vi "Test MQTT-3.8.3-3.vi"(8 "error in (no error)":errorcluster) -> (0 "error out":errorcluster)   [LabVIEW 2013]
uses:
  source/Control Packets/SUBSCRIBE/Topic Subscription -- cluster.ctl
  source/Control Packets/ControlPacket/QualityOfService -- enum.ctl
  source/Control Packets/ControlPacket/ControlPacket.lvclass/ControlPacket.ctl
  source/Client/Client.lvclass
  <vilib>/addons/_JKI Toolkits/Caraya/classes/Test/Test.lvclass
  source/Control Packets/SUBSCRIBE/SUBSCRIBE.lvclass
  source/Control Packets/ControlPacket/ControlPacket.lvclass
  <vilib>/addons/_JKI Toolkits/Caraya/classes/Assert/Assert.lvclass
  source/MQTT_Base/MQTT_Base.lvclass
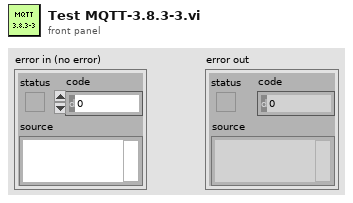
[diagram p1: front panel]
types:
  T1 = typedef "SUBSCRIBE.lvclass/Topic Subscription -- cluster.ctl" = cluster{"Topic Filter":string, "QoS":T2}
  T2 = typedef "ControlPacket.lvclass/QualityOfService -- enum.ctl" = enum16{"0 (At Most Once)", "1 (At Least Once)", "2 (Exactly Once)"}
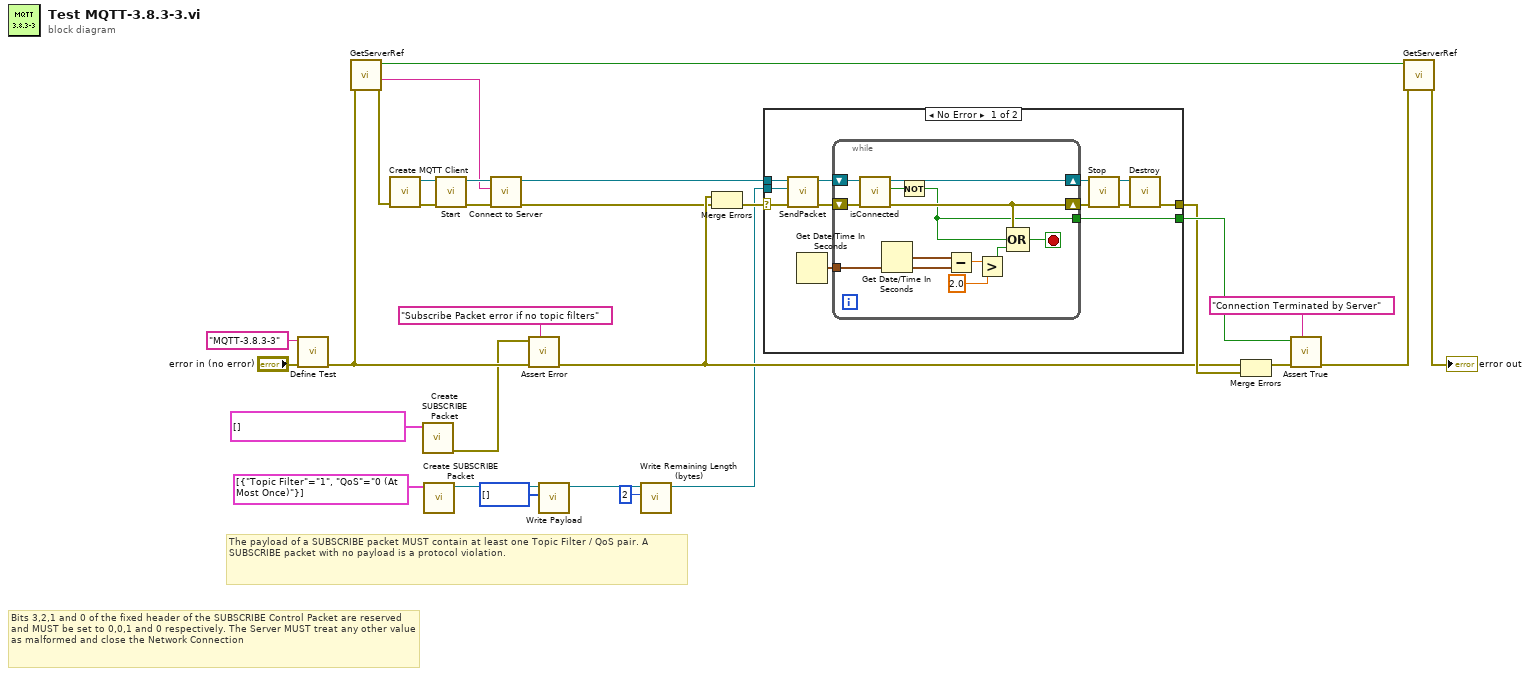
[diagram p0: block diagram]
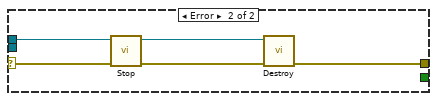
[diagram p2: hidden frame]
diagram:
  # "The payload of a SUBSCRIBE packet MUST contain at least one Topic Filter / QoS pair. A SUBSCRIBE packet with no payload is a protocol violation."
  # "Bits 3,2,1 and 0 of the fixed header of the SUBSCRIBE Control Packet are reserved and MUST be set to 0,0,1 and 0 respectively. The Server MUST treat any other value as malformed and close the Network Connection"
  n1 = call <vilib>:"Define Test.vi"("error in (no error)"="error in (no error)", "Label (VI Title)"="MQTT-3.8.3-3") -> ("error out"=w19:errorcluster)  [unwired: 9 in]
  n2 = call "GetServerRef.vi"("error in"=w19) -> ("error out"=w26:errorcluster, "Server address"=w1:string, "Created"=w27:bool)  [unwired: 7 in, 1 out]
  n3 = call "Create MQTT Client.vi"("error in (no error)"=w26) -> ("error out"=w10:errorcluster, "Client out"=w12:refnum<class "Client.lvclass">)  [unwired: 9 in]
  n4 = call "Create SUBSCRIBE Packet.vi"("Topic Subscriptions"=T1[] []) -> ("error out"=w8:errorcluster)  [unwired: 9 in, 1 out]
  n5 = call "Create SUBSCRIBE Packet.vi"("Topic Subscriptions"=T1[] [{"Topic Filter"="1", "QoS"=enum."0 (At Most Once)"}]) -> ("SUBSCRIBE out"=w6:refnum<class "SUBSCRIBE.lvclass">)  [unwired: 9 in, 1 out]
  n6 = call "Start.vi"("error in (no error)"=w10, "MQTT_Base in"=w12) -> ("error out"=w9:errorcluster, "MQTT_Base out"=w11:refnum<class "Client.lvclass">)  [unwired: 7 in, 1 out]
  n7 = call "Connect to Server.vi"("error in (no error)"=w9, "address (localhost)"=w1, "Client in"=w11) -> ("error out"=w14:errorcluster, "Client out"=w13:refnum<class "Client.lvclass">)  [unwired: 6 in, 1 out]
  n8 = call <vilib>:"Assert Error.vi"("Label"="Subscribe Packet error if no topic filters", "error in (no error)"=w19, "Error?"=w8) -> ("error out"=w16:errorcluster)  [unwired: 8 in]
  n9 = call "Write Payload.vi"("Payload"=u8[] [], "ControlPacket in"=w6) -> ("ControlPacket out"=w2:refnum<class "SUBSCRIBE.lvclass">)  [unwired: 9 in]
  n10 = call "Write Remaining Length (bytes).vi"("Remaining Length (bytes)"=u32 2, "ControlPacket in"=w2) -> ("ControlPacket out"=w4:refnum<class "SUBSCRIBE.lvclass">)  [unwired: 9 in]
  n11 = Merge Errors(w16, w14) -> (w15:errorcluster)
  n12 = case shown="No Error" w15 {
    selector: w15 -> [w39 w55]
    tunnel: w13 -> [w40 w57]
    tunnel: [w41 w58] -> w17
    tunnel: [w31 _] -> w22
    tunnel: w4 -> [w38 _]
    frame No Error {
      n13 = call "SendPacket.vi"("error in (no error)"=w39, "ControlPacket"=w38, "Client in"=w40) -> ("error out"=w34:errorcluster, "Client out"=w35:refnum<class "Client.lvclass">)  [unwired: 6 in, 1 out]
      n14 = Get Date/Time In Seconds() -> (seconds since 1Jan1904=w30:timestamp)
      n15 = while {
        shift-right: [w50] -> w33
        shift-left: w34 -> [w51]
        shift-right: [w52] -> w32
        shift-left: w35 -> [w53]
        tunnel: [w47] -> w31
        tunnel: w30 -> [w42]
        stop <- w49 stop-if-true
        n16 = call "isConnected.vi"("error in (no error)"=w51, "Client in"=w53) -> ("error out"=w50:errorcluster, "connected"=w48:bool, "Client out"=w52:refnum<class "Client.lvclass">)  [unwired: 7 in]
        n17 = Get Date/Time In Seconds() -> (seconds since 1Jan1904=w43:timestamp)
        n18 = Not(x=w48) -> (.not. x?=w47:bool)
        n19 = Subtract(x=w43, y=w42) -> (x-y=w46:dbl)
        n20 = Greater?(x=w46, y=2.0) -> (0:w44:bool)
        n21 = Compound Arithmetic op=OR(w50, w47, w44) -> (w49:bool)
      }
      n22 = call "Stop.vi"("error in (no error)"=w33, "MQTT_Base in"=w32) -> ("error out"=w36:errorcluster, "MQTT_Base out"=w37:refnum<class "Client.lvclass">)  [unwired: 7 in, 1 out]
      n23 = call-dynamic "Destroy.vi"("error in (no error)"=w36, "Client in"=w37) -> ("error out"=w41:errorcluster)  [unwired: 8 in, 1 out]
    }
    frame Error {
      n24 = call "Stop.vi"("error in (no error)"=w55, "MQTT_Base in"=w57) -> ("error out"=w54:errorcluster, "MQTT_Base out"=w56:refnum<class "Client.lvclass">)  [unwired: 7 in, 1 out]
      n25 = call-dynamic "Destroy.vi"("error in (no error)"=w54, "Client in"=w56) -> ("error out"=w58:errorcluster)  [unwired: 8 in, 1 out]
    }
  }
  n26 = Merge Errors(w16, w17) -> (w18:errorcluster)
  n27 = call <vilib>:"Assert True.vi"("Label"="Connection Terminated by Server", "error in (no error)"=w18, "True?"=w22) -> ("error out"=w25:errorcluster)  [unwired: 8 in]
  n28 = call "GetServerRef.vi"("error in"=w25, "Destroy (F)"=w27) -> ("error out"=→"error out":errorcluster)  [unwired: 6 in, 3 out]
